vi "Login Main.vi"() -> ()   [LabVIEW 2022 SP3]
uses:
  Login Case.ctl
panel:
  out "array 2":dbl[][](array[numeric])
  in  "file path (use dialog)":path
  out "array":string[][](array[string])
  in  "Select User":u16(ring) items=["Vigneshwaran", "Sarfaraz", "Parikshit", "Ajai", "Kannan", "Lingesh", "Saravana", "Mowlisa"]
  in  "Password":string
  in  "Show Password":bool
  in  "Change Password":bool
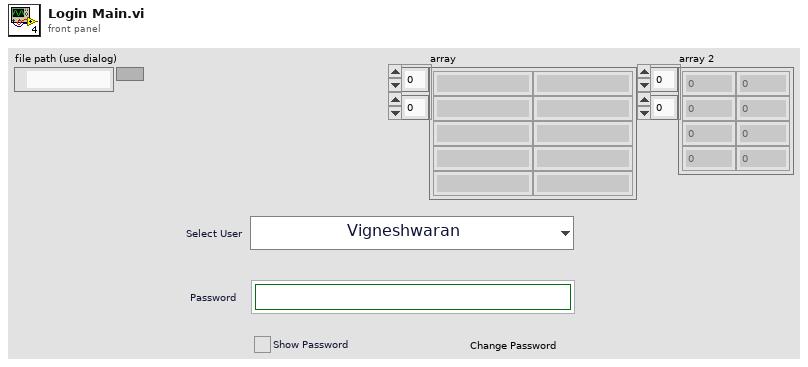
[diagram p1: front panel]
types:
  T1 = typedef "Login Case.ctl" = enum16{"Initialize", "Pole Event", "Login", "Forgot Password", "Change Password", "Exit"}
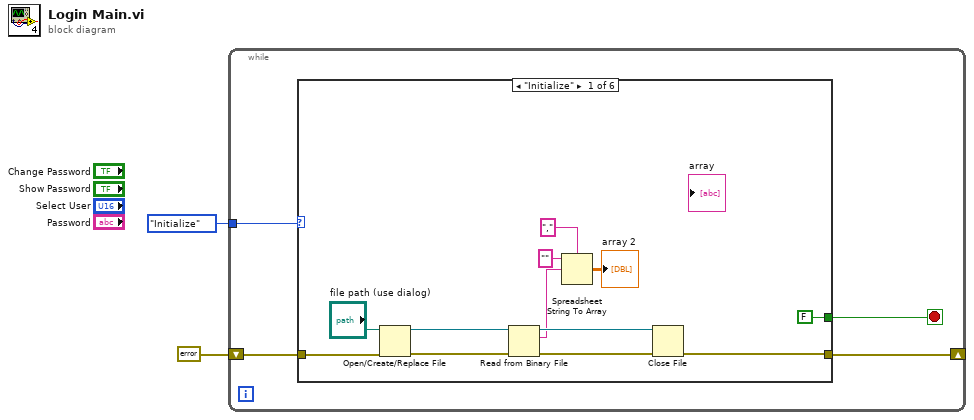
[diagram p0: block diagram]
diagram:
  n1 = while {
    tunnel: Login_Case."Initialize" -> [w6]
    shift-right: [w3] -> _
    shift-left: errorcluster {"status"=FALSE, "code"=0, "source"=""} ("error in (no error)") -> [w4]
    stop <- w5 stop-if-true
    n2 = case shown="\"Initialize\"" w6 {
      tunnel: [FALSE _ _ _ _ _] -> w5
      tunnel: w4 -> [w17 w19 w20 w21 w22 w23]
      tunnel: [w12 w19 w20 w21 w22 w23] -> w3
      frame "Initialize" {
        n3 = Open/Create/Replace File(file path (use dialog)="file path (use dialog)", error in=w17) -> (refnum out=w13:refnum<file>, error out=w16:errorcluster)  [unwired: 4 in, 1 out]
        n4 = Read from Binary File(8:w16, 11:w13) -> (0:w15:errorcluster, 2:w10:string, 3:w14:refnum<file>)  [unwired: 4 in, 1 out]
        n5 = Spreadsheet String To Array(delimiter (Tab)=",", format string="", spreadsheet string=w10) -> (array=→"array 2":dbl[][])  [unwired: 1 in]
        n6 = Close File(refnum=w14, error in=w15) -> (error out=w12:errorcluster)  [unwired: 1 out]
      }
      frame "Pole Event", Default {
      }
      frame "Login" {
      }
      frame "Forgot Password" {
      }
      frame "Change Password" {
      }
      frame "Exit" {
      }
    }
  }
